vi "A170316-11-Login.vi"() -> ()   [LabVIEW 2020]
uses:
  Database/Global1.vi
  <vilib>/addons/database/Connection.llb/DB Tools Open Connec (String).vi
  <vilib>/addons/database/Connection.llb/Conn Execute.vi
  <vilib>/addons/database/Recordset.llb/Rec Fetch Recordset Data (R).vi
  <vilib>/addons/database/NI_Database_API.lvlib
  <vilib>/addons/database/Recordset.llb/Rec Destroy - Connection.vi
panel:
  in  "登陆":bool
  in  "密   码":string
  out "数据库连接成功":bool
  in  "联机模式":enum16{"单机", "联网"}(ring)
  in  "用户名":string
  # "数据库状态"
  # "调节机构装配"
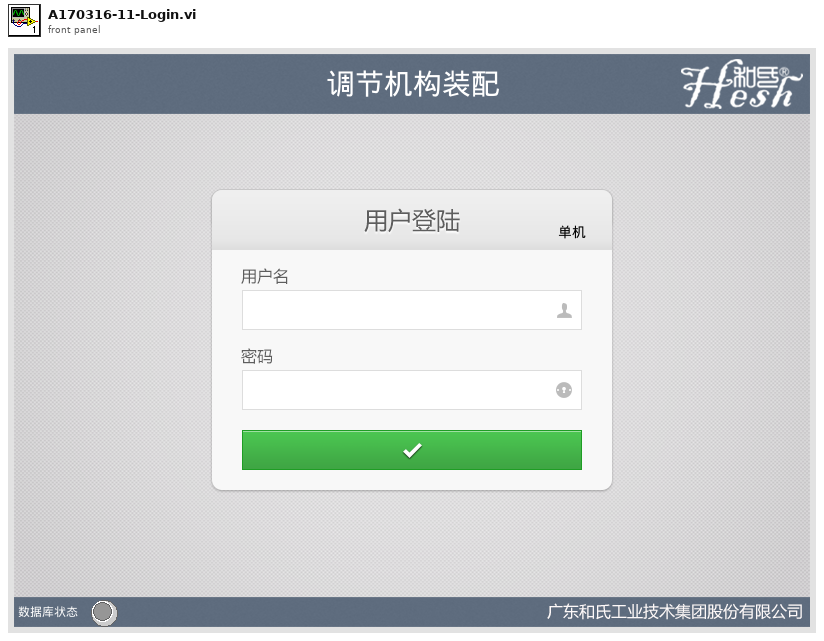
[diagram p1: front panel]
types:
  T1 = enum32{"Invalid", "Standard", "Closed", "Hidden", "Minimized", "Maximized"}
  T2 = cluster{"data[0]":string, "data[1]":string, "data[2]":string, "data[3]":string}
  T3 = typedef "NI_Database_API.lvlib/Conn ObjectReference.ctl" = refnum<k1>
  T4 = typedef "NI_Database_API.lvlib/Rec ObjectReference.ctl" = refnum<k1>
  T5 = typedef "eventvkey.ctl" = enum16{"ASCII", "Enter", "Return", "Shift", "Ctrl", "Alt", "Cmd", "Opt", "Caps", "NumLock", "Clear", "Break", "Up", "Down", "Left", "Right", "Insert", "Delete", "Home", "End", "PageUp", "PageDown", "Escape", "Help", "Pause", "ScrollLock", "F1", "F2", "F3", "F4", "F5", "F6", "F7", "F8", "F9", "F10", "F11", "F12", "F13", "F14", "F15", "F16", "F17", "F18", "F19", "F20", "F21", "F22", "F23", "F24", "Play", "VolumeUp", "VolumeDown", "Mute", "Two Byte Char"}
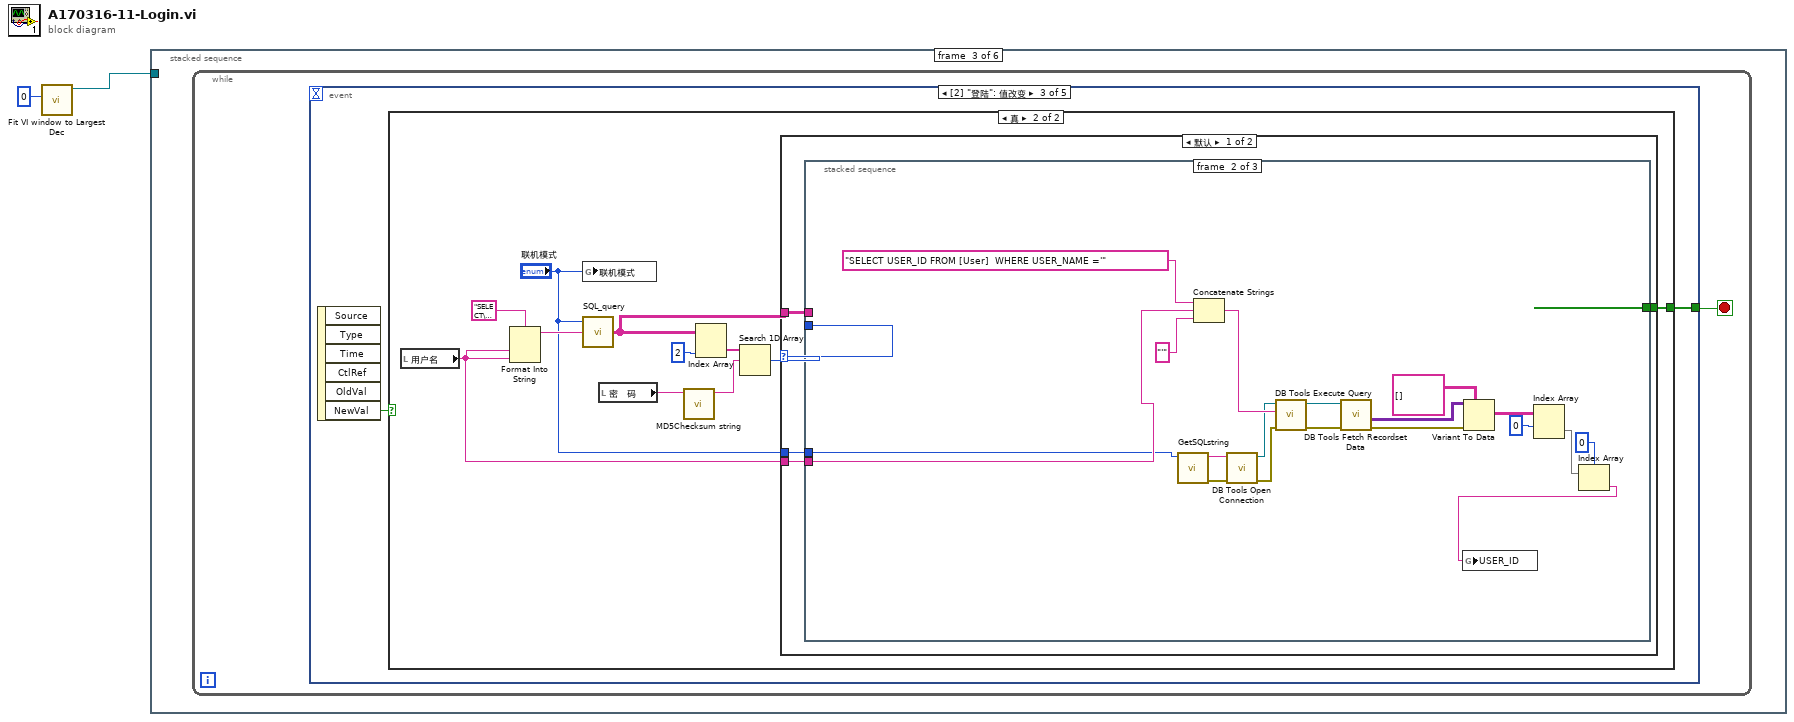
[diagram p0: block diagram]
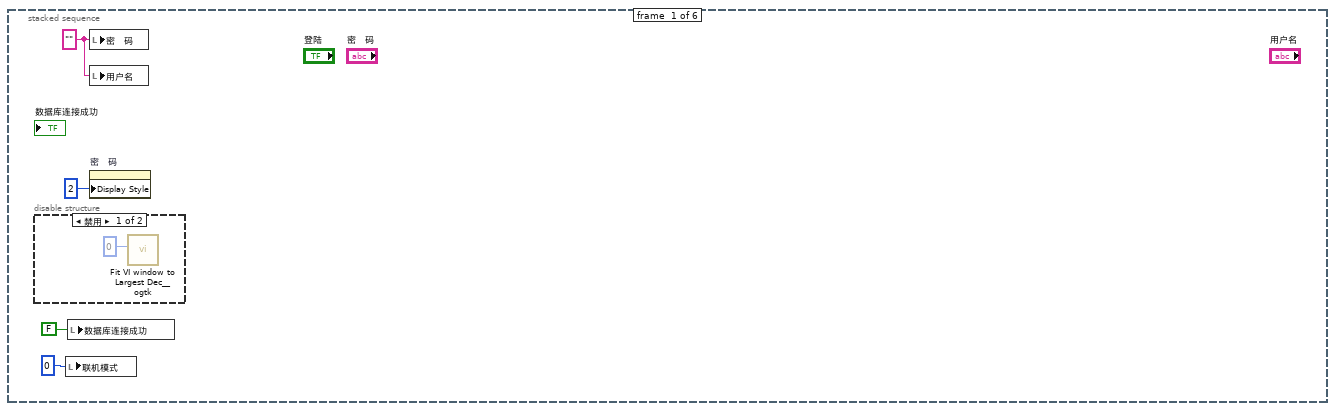
[diagram p2: hidden frame]
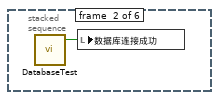
[diagram p4: hidden frame]
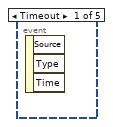
[diagram p5: hidden frame]
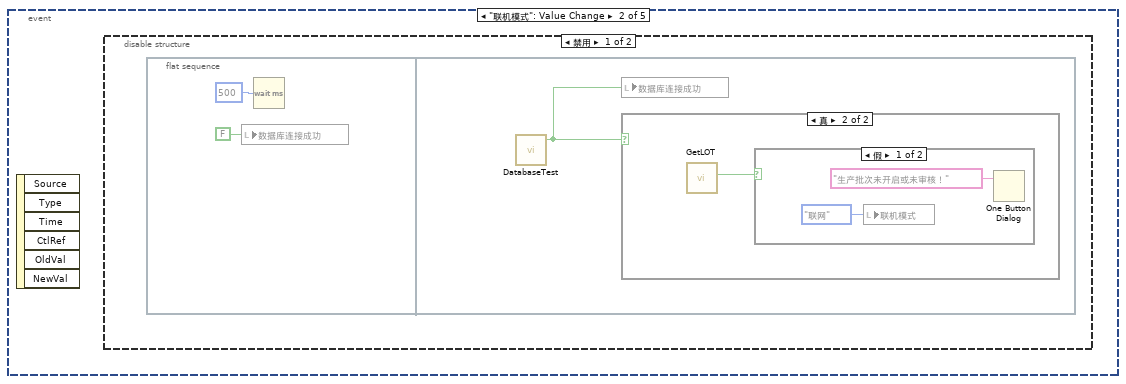
[diagram p6: hidden frame]
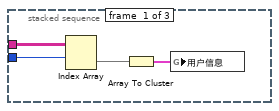
[diagram p11: hidden frame]
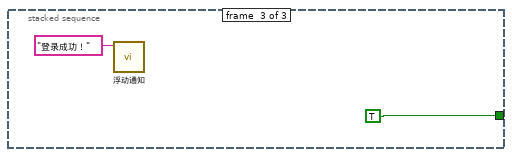
[diagram p12: hidden frame]
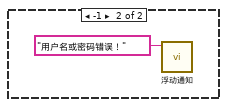
[diagram p13: hidden frame]
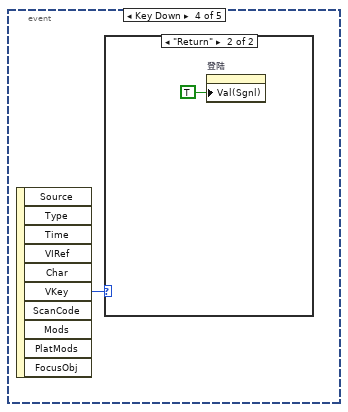
[diagram p14: hidden frame]
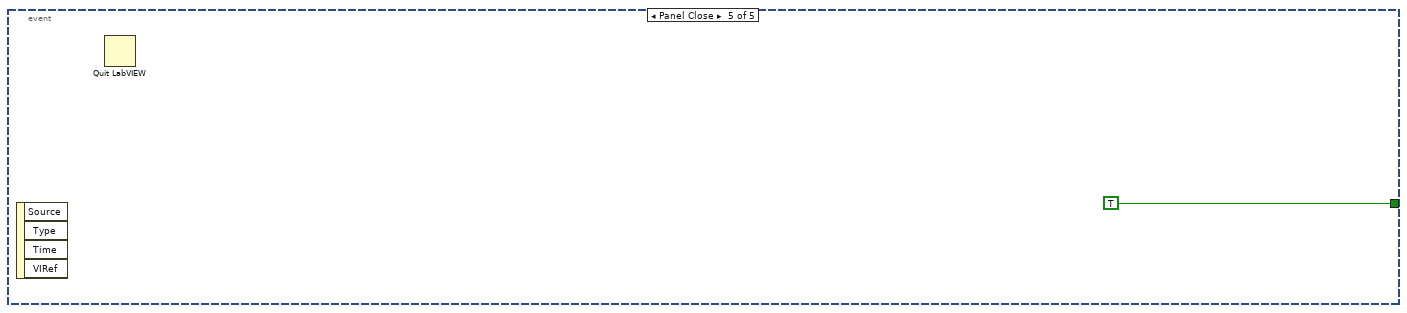
[diagram p16: hidden frame]
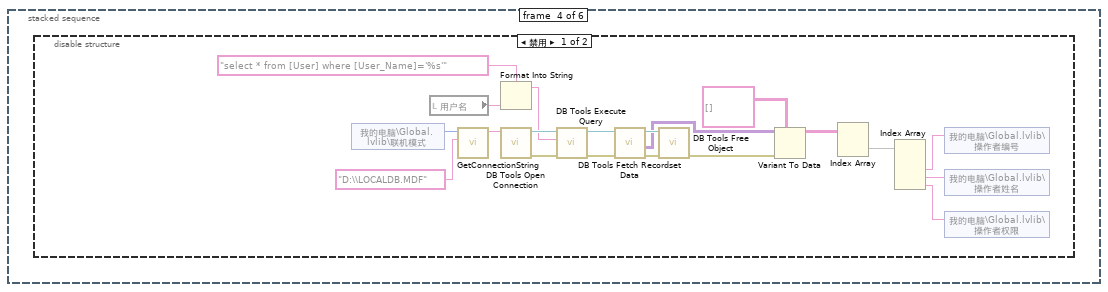
[diagram p17: hidden frame]
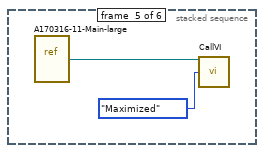
[diagram p19: hidden frame]
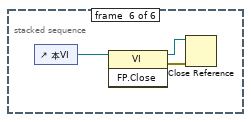
[diagram p20: hidden frame]
diagram:
  n1 = call "Fit VI window to Largest Dec.vi"("border spacing (2 px)"=0) -> ("dup VI Ref"=w1:refnum<vi>)  [unwired: 5 in, 1 out]
  n2 = stacked-sequence {
    tunnel: w1 -> [_ _ _ _ _ _]
    frame #0 {
      w4 = ""
      n3 = disable-structure shown="禁用" {
        frame Disabled {
          n4 = call <userlib>:"Fit VI window to Largest Dec__ogtk.vi"("border spacing (2 px)"=0) -> ()  [unwired: 5 in, 2 out]
        }
        frame Enabled {
        }
      }
      n5 = local write "联机模式"(u16 0 ("程序版本")) -> ()
      n6 = local write "数据库连接成功"(FALSE ("数据库连接成功")) -> ()
      n7 = local write "密   码"(w4) -> ()
      n8 = local write "用户名"(w4) -> ()
      n9 = property on="密   码" class="Str"("Display Style"=u32 2 ("显示样式")) -> ()  [unwired: 2 in, 2 out]
    }
    frame #1 {
      n10 = call "DatabaseTest.vi"() -> ("数据库连接成功"=w8:bool)  [unwired: 4 in, 1 out]
      n11 = local write "数据库连接成功"(w8) -> ()
    }
    frame #2 {
      n12 = while {
        stop <- w9 stop-if-true
        n13 = event shown="[2] \"登陆\": 值改变" {
          selector: _ -> [_ _ _ _ _]
          dyn-events: _ -> [_ _ _ _ _]
          timeout: _ -> [_ _ _ _ _]
          tunnel: [_ _ w16 _ TRUE] -> w9
          event Timeout {
            n14 = event-data() -> ()  [unwired: 1 in, 3 out]
          }
          event "联机模式": Value Change {
            n15 = event-data() -> ()  [unwired: 1 in, 6 out]
            n16 = disable-structure shown="禁用" {
              frame Disabled {
                n17 = flat-sequence {
                  frame #0 {
                    n18 = local write "数据库连接成功"(FALSE ("数据库连接成功")) -> ()
                    n19 = Wait (ms)(milliseconds to wait=u32 500 ("等待时间（毫秒）")) -> ()  [unwired: 1 out]
                  }
                  frame #1 {
                    n20 = call "DatabaseTest.vi"() -> ("数据库连接成功"=w12:bool)  [unwired: 4 in, 1 out]
                    n21 = local write "数据库连接成功"(w12) -> ()
                    n22 = case shown="真" w12 {
                      frame False {
                      }
                      frame True {
                        n23 = call "GetLOT.vi"() -> ("生产批次有效"=w13:bool)  [unwired: 9 in, 2 out]
                        n24 = case shown="假" w13 {
                          frame False {
                            n25 = local write "联机模式"(enum16{"单机", "联网"}."联网" ("联机模式")) -> ()
                            n26 = One Button Dialog(message="生产批次未开启或未审核！" ("消息")) -> ()  [unwired: 1 in, 1 out]
                          }
                          frame True {
                          }
                        }
                      }
                    }
                  }
                }
              }
              frame Enabled {
              }
            }
          }
          event "登陆": Value Change {
            n27 = event-data() -> ("NewVal"=w17:bool)  [unwired: 1 in, 5 out]
            n28 = case shown="真" w17 {
              tunnel: [_ w20] -> w16
              frame False {
              }
              frame True {
                n29 = local read "用户名"() -> (w19:string)
                n30 = Format Into String(format string="SELECT\ndbo.[User].USER_EMPLOYEE_ID,\ndbo.[User].USER_NAME,\ndbo.[User].USER_PASSWD,\ndbo.[User].USER_PERMIT\n\nFROM\ndbo.[User]\nWHERE\ndbo.[User].USER_NAME = '%s' \nOR\ndbo.[User].USER_EMPLOYEE_ID = '%s'\n" ("格式字符串"), w19, w19) -> (resulting string=w26:string)  [unwired: 2 in, 1 out]
                n31 = global write "Global1.vi" "联机模式"("联机模式") -> ()
                n32 = call "SQL_query.vi"("SQL query"=w26, "联机模式"="联机模式") -> ("data"=w21:string[][])  [unwired: 1 in, 2 out]
                n33 = local read "密   码"() -> (w28:string)
                n34 = call <vilib>:"MD5Checksum string.vi"("Message String"=w28) -> ("MD5 message-digest"=w22:string)  [unwired: 10 in]
                n35 = Index Array(array=w21, index (col)=2 ("禁用的索引 (列)")) -> (element=w25:string[])  [unwired: 1 in]
                n36 = Search 1D Array(1D array=w25, element=w22) -> (index of element=w23:i32)  [unwired: 1 in]
                n37 = case shown="默认" w23 {
                  selector: w23 -> [w33 _]
                  tunnel: w21 -> [w32 _]
                  tunnel: [w31 _] -> w20
                  tunnel: w19 -> [w30 _]
                  tunnel: "联机模式" -> [w29 _]
                  frame Default {
                    n38 = stacked-sequence {
                      tunnel: w33 -> [w34 _ _]
                      tunnel: w32 -> [w36 _ _]
                      tunnel: [_ _ TRUE] -> w31
                      tunnel: w30 -> [_ w40 _]
                      tunnel: w29 -> [_ w39 _]
                      frame #0 {
                        n39 = Index Array(array=w36, index (row)=w34) -> (element=w35:string[])  [unwired: 1 in]
                        n40 = Array To Cluster(array=w35) -> (cluster=w37:T2)
                        n41 = global write "Global1.vi" "用户信息"(w37) -> ()
                      }
                      frame #1 {
                        n42 = call "GetSQLstring.vi"("联机模式"=w39) -> ("错误输出"=w55:errorcluster, "连接字符串"=w56:string)  [unwired: 9 in]
                        n43 = Concatenate Strings("SELECT USER_ID FROM [User]  WHERE USER_NAME ='" ("字符串"), w40, "'" ("字符串")) -> (w54:string)
                        n44 = call-poly <vilib>:"DB Tools Open Connection.vi"("error in (no error)"=w55, "connection information"=w56) -> ("error out"=w48:errorcluster, "connection reference"=w49:T3)  [unwired: 6 in]
                        n45 = call-poly <vilib>:"DB Tools Execute Query.vi"("error in (no error)"=w48, "SQL query"=w54, "connection reference"=w49) -> ("error out"=w52:errorcluster, "recordset reference"=w53:T4)  [unwired: 5 in]
                        n46 = call-poly <vilib>:"DB Tools Fetch Recordset Data.vi"("error in (no error)"=w52, "recordset reference"=w53) -> ("error out"=w46:errorcluster, "recordset data"=w51:variant[][])  [unwired: 3 in, 1 out]
                        n47 = Variant To Data(error in=w46, type=string[][] [], Variant=w51) -> (data=w45:string[][])  [unwired: 1 out]
                        n48 = Index Array(array=w45, index (row)=0 ("索引 (行)")) -> (element=w43:string[])  [unwired: 1 in]
                        n49 = Index Array(array=w43, index=0 ("索引 (行)")) -> (element=w38:string)
                        n50 = global write "Global1.vi" "USER_ID"(w38) -> ()
                      }
                      frame #2 {
                        n51 = call "浮动通知.vi"("通知内容"="登录成功！") -> ()  [unwired: 11 in]
                      }
                    }
                  }
                  frame -1 {
                    n52 = call "浮动通知.vi"("通知内容"="用户名或密码错误！") -> ()  [unwired: 11 in]
                  }
                }
              }
            }
          }
          event Key Down {
            n53 = event-data() -> ("VKey"=w60:T5)  [unwired: 1 in, 9 out]
            n54 = case shown="\"Return\"" w60 {
              frame "ASCII", Default {
              }
              frame "Return" {
                n55 = property on="登陆" class="Bool (严格)"("Val(Sgnl)"=TRUE ("值(信号)")) -> ()  [unwired: 2 in, 2 out]
              }
            }
          }
          event Panel Close {
            n56 = event-data() -> ()  [unwired: 1 in, 4 out]
            n57 = Quit LabVIEW() -> ()  [unwired: 1 in]
          }
        }
      }
    }
    frame #3 {
      n58 = disable-structure shown="禁用" {
        frame Disabled {
          n59 = shared-variable "我的电脑\\Global.lvlib\\联机模式"() -> (w63:i16)  [unwired: 1 in, 1 out]
          n60 = local read "用户名"() -> (w65:string)
          n61 = call "GetConnectionString.vi"("Database Name"="D:\\LOCALDB.MDF", "连接模式"=w63) -> ("连接字符串"=w81:string)  [unwired: 4 in, 1 out]
          n62 = Format Into String(format string="select * from [User] where [User_Name]='%s'", w65) -> (resulting string=w64:string)  [unwired: 2 in, 1 out]
          n63 = call-poly <vilib>:"DB Tools Open Connection.vi"("connection information"=w81) -> ("error out"=w80:errorcluster, "connection reference"=w79:T3)  [unwired: 7 in]
          n64 = call-poly <vilib>:"DB Tools Execute Query.vi"("error in (no error)"=w80, "SQL query"=w64, "connection reference"=w79) -> ("error out"=w76:errorcluster, "recordset reference"=w78:T4)  [unwired: 5 in]
          n65 = call-poly <vilib>:"DB Tools Fetch Recordset Data.vi"("error in (no error)"=w76, "recordset reference"=w78) -> ("error out"=w75:errorcluster, "recordset data"=w73:variant[][], "recordset reference out"=w77:T4)  [unwired: 3 in]
          n66 = call-poly <vilib>:"DB Tools Free Object.vi"("error in (no error)"=w75, "recordset reference"=w77) -> ("error out"=w74:errorcluster)  [unwired: 8 in, 1 out]
          n67 = Variant To Data(error in=w74, type=string[][] [], Variant=w73) -> (data=w71:string[][])  [unwired: 1 out]
          n68 = Index Array(array=w71) -> (element=w70:string[])  [unwired: 2 in]
          n69 = Index Array(array=w70) -> (element #2=w67:string, element #3=w68:string, element #4=w69:string)  [unwired: 4 in, 1 out]
          n70 = shared-variable "我的电脑\\Global.lvlib\\操作者编号"(w67) -> ()  [unwired: 1 in, 1 out]
          n71 = shared-variable "我的电脑\\Global.lvlib\\操作者姓名"(w68) -> ()  [unwired: 1 in, 1 out]
          n72 = shared-variable "我的电脑\\Global.lvlib\\操作者权限"(w69) -> ()  [unwired: 1 in, 1 out]
        }
        frame Enabled {
        }
      }
    }
    frame #4 {
      n73 = vi-ref "A170316-11-Main-large.vi"() -> (w84:refnum<vi>)
      n74 = call "CallVI.vi"("VI引用"=w84, "状态"=T1."Maximized") -> ()  [unwired: 11 in, 3 out]
    }
    frame #5 {
      n75 = control-ref of="本VI"() -> (w85:refnum<vi>)
      n76 = invoke class="VI" method="FP.Close"(reference=w85) -> (reference out=w86:refnum<vi>, error out=w87:errorcluster)  [unwired: 2 in, 1 out]
      n77 = Close Reference(reference=w86, error in (no error)=w87) -> ()  [unwired: 1 out]
    }
  }
